vi "Read and Write Channel Values.vi"(6 "Compiled.Settings":T1, 8 "error in":errorcluster, 9 "Inputs Reference in":T3, 10 "Outputs Reference in":T4, 11 "Status Reference in":T4) -> (0 "error out":errorcluster)   [LabVIEW 2019, in "Profile Interpolation Engine.lvlib"]
uses:
  Profile Interpolation Engine.lvlib
  <vilib>/NI/NIVS Inline Async API/_Data Access Engine/Data Access Engine/Types/Write.DVR.ctl
  <vilib>/NI/NIVS Inline Async API/_Data Access Engine/Access Type Classes/Write/Write.lvclass
  <vilib>/NI/NIVS Inline Async API/_Data Access Engine/Data Access Engine/Types/Read.DVR.ctl
  <vilib>/NI/NIVS Inline Async API/_Data Access Engine/Access Type Classes/Read/Read.lvclass
  Shared/Types/Compiled.Settings.ctl
  <vilib>/NI VeriStand/Custom Device API/Custom Device Target Type.ctl
  <vilib>/NI/NIVS Inline Async API/_Data Access Engine/Access Type Classes/Read/Read.lvclass/Read.ctl
  <vilib>/NI/NIVS Inline Async API/_Data Access Engine/Access Type Classes/Write/Write.lvclass/Write.ctl
  <vilib>/NI/NIVS Inline Async API/_Data Access Engine/Data Access Engine/Methods/Read.Data.vi
  <vilib>/NI/NIVS Inline Async API/_Data Access Engine/Data Access Engine/Methods/Write.Data.vi
  <vilib>/NI/NIVS Inline Async API/_Data Access Engine/Access Type Classes/Read/Read.ProcessData.vi
  <vilib>/NI/NIVS Inline Async API/_Data Access Engine/Access Type Classes/Write/Write.ProcessData.vi
  <vilib>/NI/NIVS Inline Async API/_Data Access Engine/Data Access Engine/Data Access Engine.lvclass
  Shared/Profile Interpolation Shared.lvlib
  <vilib>/NI VeriStand/Custom Device API/Custom Device API.lvlib
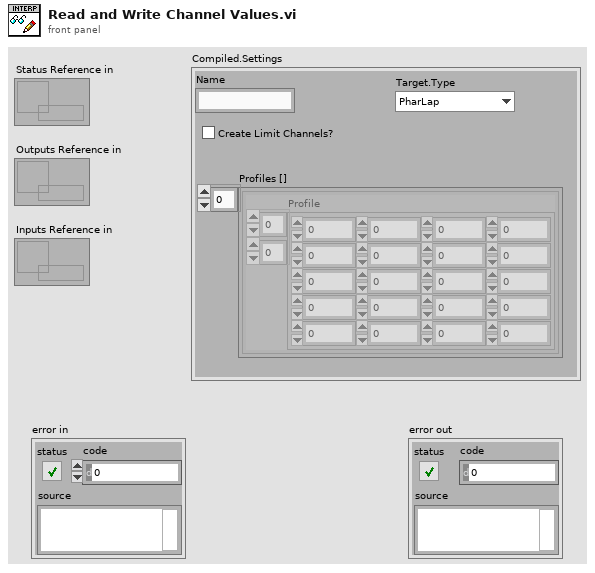
[diagram p1: front panel]
types:
  T1 = typedef "Profile Interpolation Shared.lvlib/Compiled.Settings.ctl" = cluster{"Name":string, "Create Limit Channels?":bool, "Profiles []":cluster{"Profile":dbl[][]}[], "Target.Type":T2}
  T2 = typedef "Custom Device API.lvlib/Custom Device Target Type.ctl" = enum16{"PharLap", "VxWorks", "Windows", "Linux_32_ARM", "Linux_x64"}
  T3 = typedef "Data Access Engine.lvlib/Data Access Engine.lvclass/Read.DVR.ctl" = refnum<data-value>
  T4 = typedef "Data Access Engine.lvlib/Data Access Engine.lvclass/Write.DVR.ctl" = refnum<data-value>
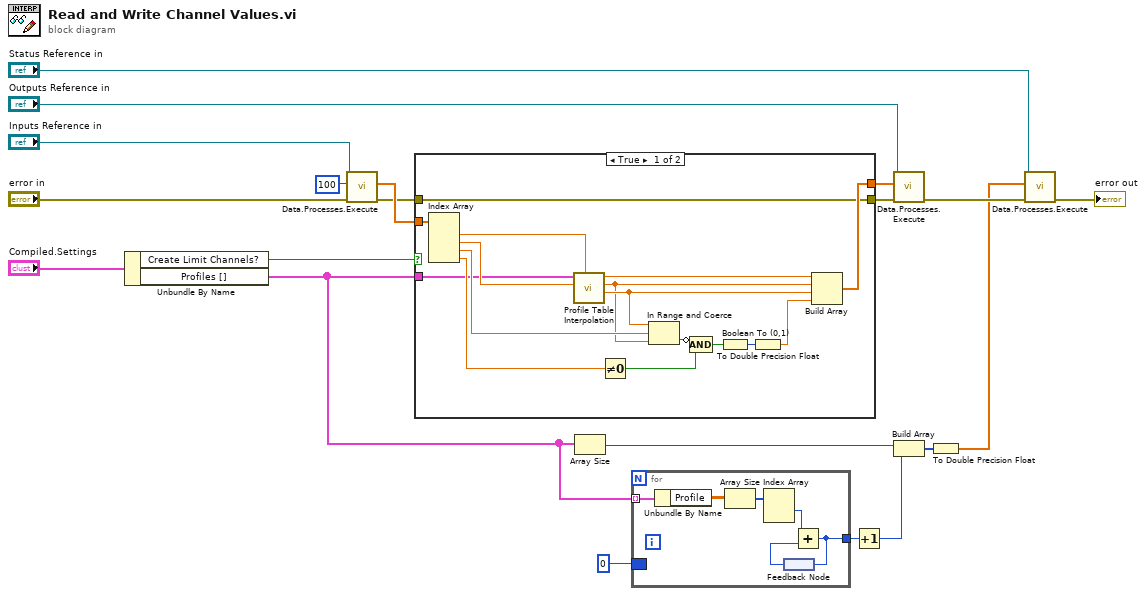
[diagram p0: block diagram]
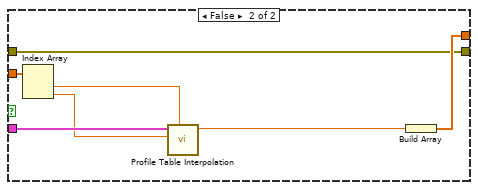
[diagram p2: hidden frame]
diagram:
  n1 = Unbundle By Name("Compiled.Settings") -> ("Create Limit Channels?"=w8:bool, "Profiles []"=w7:cluster{"Profile":dbl[][]}[])
  n2 = call-poly <vilib>:"Data.Processes.Execute.vi"("error in (no error)"="error in", "timeout ms"=100, "Ref"="Inputs Reference in") -> ("error out"=w9:errorcluster, "Values"=w12:dbl[])  [unwired: 6 in, 1 out]
  n3 = case shown="True" w8 {
    tunnel: w12 -> [w36 w43]
    tunnel: w7 -> [w22 w42]
    tunnel: [w34 w39] -> w11
    tunnel: [w24 w37] -> w10
    tunnel: w9 -> [w24 w37]
    frame True {
      n4 = Index Array(array=w36) -> (element #1=w23:dbl, element #2=w35:dbl, element #3=w33:dbl, element #4=w28:dbl)  [unwired: 4 in]
      n5 = call "Profile Table Interpolation.vi"("Profile Select"=w23, "x"=w35, "Profiles []"=w22) -> ("Interpolated y-MaxLimit"=w32:dbl, "Interpolated y-MinLimit"=w30:dbl, "Interpolated y"=w31:dbl)  [unwired: 5 in, 1 out]
      n6 = Not Equal To 0?(x=w28) -> (x != 0?=w27:bool)
      n7 = In Range and Coerce(upper limit=w32, x=w33, lower limit=w30) -> (In Range?=w29:bool)  [unwired: 1 out]
      n8 = Compound Arithmetic op=AND(invert w29, w27) -> (w26:bool)
      n9 = Boolean To (0,1)(Boolean=w26) -> (0, 1=w25:i16)
      n10 = To Double Precision Float(number=w25) -> (double precision float=w21:dbl)
      n11 = Build Array(w31, w30, w32, w21) -> (w34:dbl[])
    }
    frame False {
      n12 = Index Array(array=w43) -> (element #1=w40:dbl, element #2=w41:dbl)  [unwired: 2 in]
      n13 = call "Profile Table Interpolation.vi"("Profile Select"=w40, "x"=w41, "Profiles []"=w42) -> ("Interpolated y"=w38:dbl)  [unwired: 5 in, 3 out]
      n14 = Build Array(w38) -> (w39:dbl[])
    }
  }
  n15 = Array Size(array=w7) -> (size(s)=w6:i32)
  n16 = for {
    tunnel: w7 -> [w49] mode=indexing
    tunnel: [w44] -> w2
    border: 0 ("element") -> [_]
    n17 = Unbundle By Name(w49) -> ("Profile"=w48:dbl[][])
    n18 = Array Size(array=w48) -> (size(s)=w47:i32[])
    n19 = Index Array(array=w47) -> (element #1=w46:i32)  [unwired: 2 in, 1 out]
    n20 = feedback #1() -> (w45:i32)
    n21 = Add(x=w46, y=w45) -> (x+y=w44:i32)
    n22 = feedback-in #1(w44) -> ()
  }
  n23 = Increment(x=w2) -> (x+1=w1:i32)
  n24 = call-poly <vilib>:"Data.Processes.Execute.vi"("error in (no error)"=w10, "Values"=w11, "Ref"="Outputs Reference in") -> ("error out"=w14:errorcluster)  [unwired: 8 in]
  n25 = Build Array(w6, w1) -> (w5:i32[])
  n26 = To Double Precision Float(number=w5) -> (double precision float=w4:dbl[])
  n27 = call-poly <vilib>:"Data.Processes.Execute.vi"("error in (no error)"=w14, "Values"=w4, "Ref"="Status Reference in") -> ("error out"=→"error out":errorcluster)  [unwired: 8 in]
